vi "Evaluate (Array).vi"(8 "error in (no error)":errorcluster, 10 "Trigger Data":dbl[](array[numeric]), 11 "Trigger in":refnum<class "Trigger.lvclass">) -> (0 "error out":errorcluster, 2 "Trigger":bool, 3 "Trigger out":refnum<class "Trigger.lvclass">)   [LabVIEW 2012, in "Waveform Data Logger Engine.lvlib" / "Trigger.lvclass"]
doc: "Evaluates the trigger data and returns whether the specified trigger condition was met."
uses:
  Trigger.lvclass
  Trigger.lvclass/Trigger.ctl
  Digital Edge Trigger/Digital Edge Trigger.lvclass
  Analog Edge Trigger/Analog Edge Trigger.lvclass
  Value Change Trigger/Value Change Trigger.lvclass
  Boolean Evaluation Trigger/Boolean Evaluation Trigger.lvclass
  In Range Trigger/In Range Trigger.lvclass
  Default Trigger/Default Trigger.lvclass
panel:
  out "Trigger indices":i32[](array[numeric])
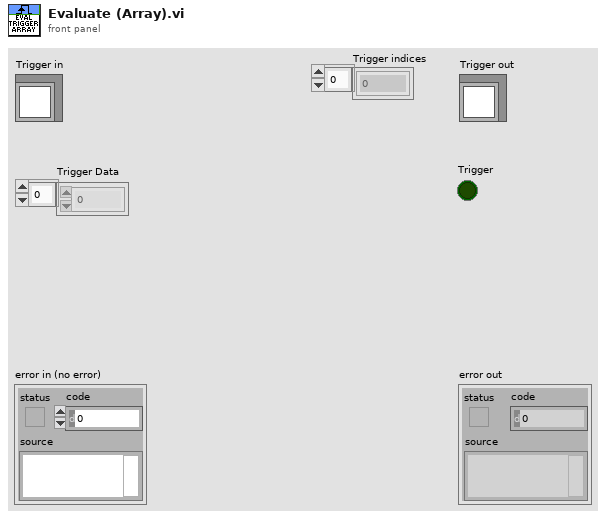
[diagram p1: front panel]
types:
  T1 = typedef "Waveform Data Logger Engine.lvlib/Trigger.lvclass/Trigger Type.ctl" = enum16{"Default", "Digital Edge", "Analog Edge", "In Range", "Value Change", "Boolean Evaluation"}
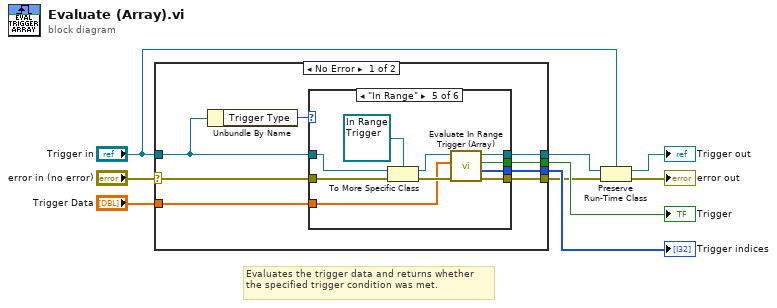
[diagram p0: block diagram]
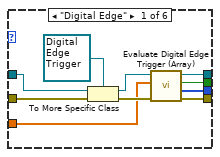
[diagram p2: hidden frame]
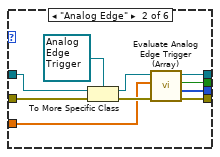
[diagram p3: hidden frame]
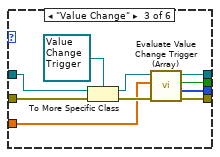
[diagram p4: hidden frame]
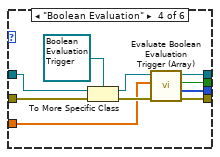
[diagram p5: hidden frame]
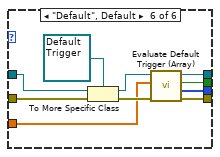
[diagram p6: hidden frame]
diagram:
  # "Evaluates the trigger data and returns whether the specified trigger condition was met."
  n1 = case shown="No Error" "error in (no error)" {
    selector: "error in (no error)" -> [w14 w78]
    tunnel: "Trigger in" -> [w16 w79]
    tunnel: [w15 w79] -> w3
    tunnel: [w13 w78] -> w5
    tunnel: "Trigger Data" -> [w12 _]
    tunnel: [w11 _] -> w7
    tunnel: [w10 _] -> w6
    frame No Error {
      n2 = Unbundle By Name(w16) -> ("Trigger Type"=w17:T1)
      n3 = case shown="\"In Range\"" w17 {
        tunnel: w16 -> [w25 w37 w47 w57 w67 w77]
        tunnel: [w27 w31 w41 w51 w61 w71] -> w15
        tunnel: [w22 w33 w43 w53 w63 w73] -> w13
        tunnel: w14 -> [w21 w36 w46 w56 w66 w76]
        tunnel: w12 -> [w20 w30 w40 w50 w60 w70]
        tunnel: [w19 w29 w39 w49 w59 w69] -> w11
        tunnel: [w18 w28 w38 w48 w58 w68] -> w10
        frame "Digital Edge" {
          n4 = To More Specific Class(target class=refnum<class "Digital Edge Trigger.lvclass"> refnum ("Digital Edge Trigger.lvclass"), reference=w25, error in=w21) -> (specific class reference=w23:refnum<class "Digital Edge Trigger.lvclass">, error out=w26:errorcluster)
          n5 = call "Evaluate Digital Edge Trigger (Array).vi"("error in (no error)"=w26, "Trigger Data"=w20, "Digital Edge Trigger in"=w23) -> ("error out"=w22:errorcluster, "Trigger indices"=w18:i32[], "Trigger"=w19:bool, "Digital Edge Trigger out"=w27:refnum<class "Digital Edge Trigger.lvclass">)  [unwired: 5 in]
        }
        frame "Analog Edge" {
          n6 = To More Specific Class(target class=refnum<class "Analog Edge Trigger.lvclass"> refnum ("Analog Edge Trigger.lvclass"), reference=w37, error in=w36) -> (specific class reference=w32:refnum<class "Analog Edge Trigger.lvclass">, error out=w34:errorcluster)
          n7 = call "Evaluate Analog Edge Trigger (Array).vi"("error in (no error)"=w34, "Trigger Data"=w30, "Analog Edge Trigger in"=w32) -> ("error out"=w33:errorcluster, "Trigger indices"=w28:i32[], "Trigger"=w29:bool, "Analog Edge Trigger out"=w31:refnum<class "Analog Edge Trigger.lvclass">)  [unwired: 5 in]
        }
        frame "Value Change" {
          n8 = To More Specific Class(target class=refnum<class "Value Change Trigger.lvclass"> refnum ("Value Change Trigger.lvclass"), reference=w47, error in=w46) -> (specific class reference=w42:refnum<class "Value Change Trigger.lvclass">, error out=w44:errorcluster)
          n9 = call "Evaluate Value Change Trigger (Array).vi"("error in (no error)"=w44, "Trigger Data"=w40, "Value Change Trigger in"=w42) -> ("error out"=w43:errorcluster, "Trigger indices"=w38:i32[], "Trigger"=w39:bool, "Value Change Trigger out"=w41:refnum<class "Value Change Trigger.lvclass">)  [unwired: 5 in]
        }
        frame "Boolean Evaluation" {
          n10 = To More Specific Class(target class=refnum<class "Boolean Evaluation Trigger.lvclass"> refnum ("Boolean Evaluation Trigger.lvclass"), reference=w57, error in=w56) -> (specific class reference=w52:refnum<class "Boolean Evaluation Trigger.lvclass">, error out=w54:errorcluster)
          n11 = call "Evaluate Boolean Evaluation Trigger (Array).vi"("error in (no error)"=w54, "Trigger Data"=w50, "Boolean Evaluation Trigger in"=w52) -> ("error out"=w53:errorcluster, "Trigger indices"=w48:i32[], "Trigger"=w49:bool, "Boolean Evaluation Trigger out"=w51:refnum<class "Boolean Evaluation Trigger.lvclass">)  [unwired: 5 in]
        }
        frame "In Range" {
          n12 = To More Specific Class(target class=refnum<class "In Range Trigger.lvclass"> refnum ("In Range Trigger.lvclass"), reference=w67, error in=w66) -> (specific class reference=w62:refnum<class "In Range Trigger.lvclass">, error out=w64:errorcluster)
          n13 = call "Evaluate In Range Trigger (Array).vi"("error in (no error)"=w64, "Trigger Data"=w60, "In Range Trigger in"=w62) -> ("error out"=w63:errorcluster, "Trigger indices"=w58:i32[], "Trigger"=w59:bool, "In Range Trigger out"=w61:refnum<class "In Range Trigger.lvclass">)  [unwired: 5 in]
        }
        frame "Default", Default {
          n14 = To More Specific Class(target class=refnum<class "Default Trigger.lvclass"> refnum ("Default Trigger.lvclass"), reference=w77, error in=w76) -> (specific class reference=w72:refnum<class "Default Trigger.lvclass">, error out=w74:errorcluster)
          n15 = call "Evaluate Default Trigger (Array).vi"("error in (no error)"=w74, "Trigger Data"=w70, "Default Trigger in"=w72) -> ("error out"=w73:errorcluster, "Trigger indices"=w68:i32[], "Trigger"=w69:bool, "Default Trigger out"=w71:refnum<class "Default Trigger.lvclass">)  [unwired: 5 in]
        }
      }
    }
    frame Error {
    }
  }
  "Trigger" <- w7
  "Trigger indices" <- w6
  n16 = Preserve Run-Time Class(object in=w3, error in=w5, 2:"Trigger in") -> (object out=→"Trigger out":refnum<class "Trigger.lvclass">, error out=→"error out":errorcluster)
